vi "Check DC_X.vi"   [LabVIEW 2012, in "4134Outputs.lvlib"]
uses:
  4134Outputs.lvlib
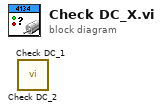
[diagram p0: block diagram]
diagram:
  n1 = call "Check DC_2.vi"() -> ()  [unwired: 11 in, 5 out]
  n2 = call "Check DC_1.vi"() -> ()  [unwired: 13 in, 3 out]
